vi "Input 信息检测.vi"(9 "Input 配置信息":string[][](table)=[["名称", "点位", "索引号", "逻辑取反"], ["启动按钮", "X100", "0", "0"], ["复位按钮", "X101", "1", "0"], ["暂停按钮", "X102", "2", "0"], ["操作侧安全光栅", "X103", "3", "0"], ["后侧安全光栅", "X104", "4", "0"], ["上层真空检知", "X105", "5", "0"], ["下层真空检知", "X106", "6", "0"], ["上层感应sensor", "X107", "7", "0"], ["下层感应sensor", "X110", "8", "0"], ["传送抓手气缸前位", "X111", "9", "0"], ["传送抓手气缸后位", "X112", "10", "0"], ["上层产品定位气缸前位", "X113", "11", "0"], ["上层产品定位气缸后位", "X114", "12", "0"], ["下层产品定位气缸前位", "X115", "13", "0"], ["下层产品定位气缸后位", "X116", "14", "0"], ["抓手感应产品sensor", "X117", "15", "0"], ["起子1真空检知", "X120", "16", "0"], ["起子2真空检知", "X121", "17", "0"], ["起子3真空检知", "X122", "18", "0"], ["起子4真空检知", "X123", "19", "0"], ["feed01感应sensor", "X124", "20", "0"], ["feed02感应sensor", "X125", "21", "0"], ["feed03感应sensor", "X126", "22", "0"], ["feed04感应sensor", "X127", "23", "0"], ["动子1和2统一坐标sensor", "X130", "24", "0"], ["动子3和4统一坐标sensor", "X131", "25", "0"], ["前后侧统一坐标sensor", "X132", "26", "0"], ["上站允许取料信号", "X133", "27", "0"], ["下站允许投料信号", "X134", "28", "0"], ["上站请求信号", "X135", "29", "0"], ["下站答复信号", "X136", "30", "0"]], 11 "输入读取":T1) -> (2 "Input  ERROR":string[](array[string]))   [LabVIEW 2017]
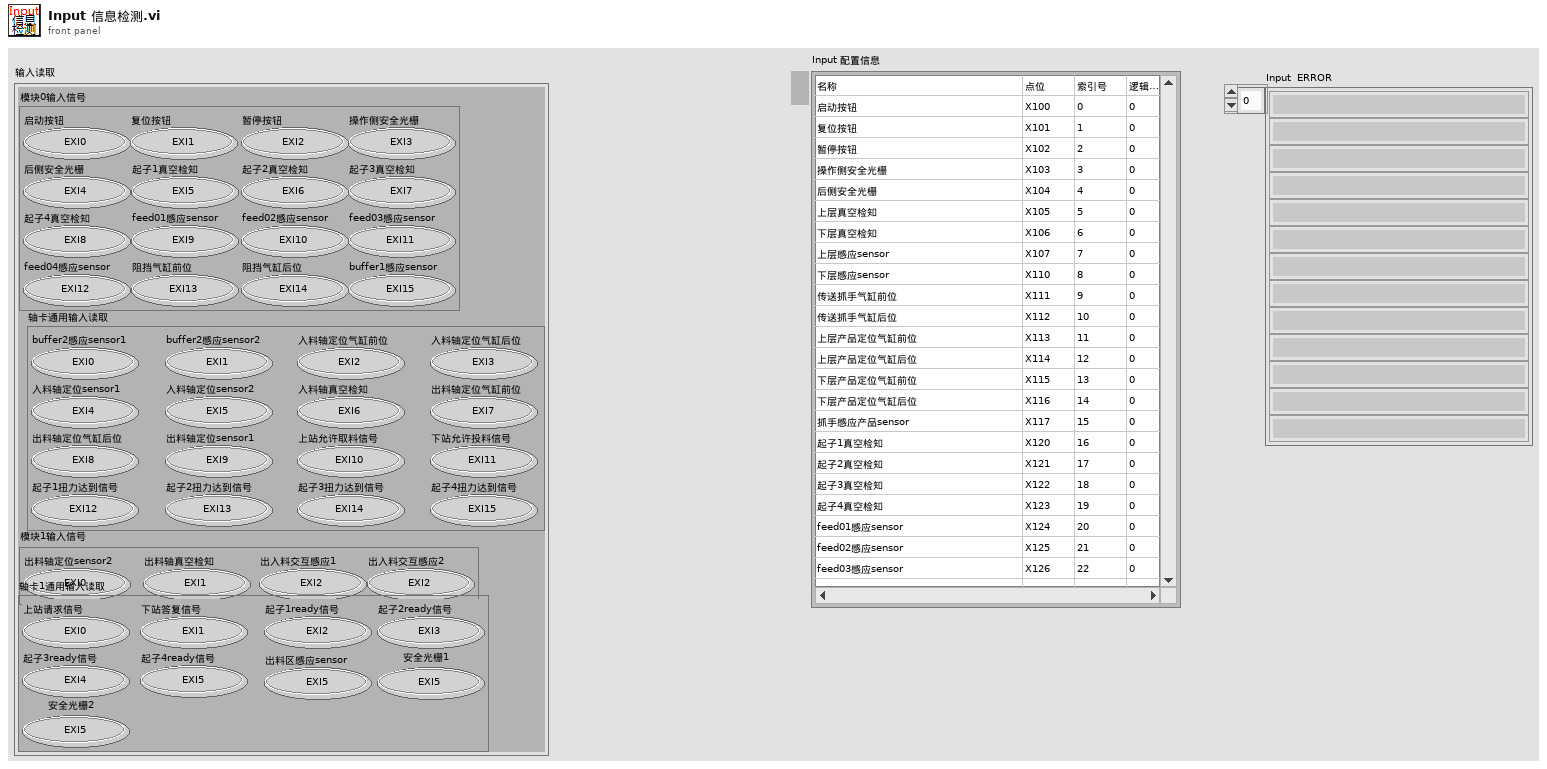
[diagram p1: front panel]
types:
  T1 = typedef "输入读取.ctl" = cluster{"模块0输入信号":T2, "轴卡通用输入读取":T3, "模块1输入信号":T4, "轴卡1通用输入读取":T5}
  T2 = typedef "模块0输入读取.ctl" = cluster{"启动按钮":bool, "复位按钮":bool, "暂停按钮":bool, "操作侧安全光栅":bool, "后侧安全光栅":bool, "起子1真空检知":bool, "起子2真空检知":bool, "起子3真空检知":bool, "起子4真空检知":bool, "feed01感应sensor":bool, "feed02感应sensor":bool, "feed03感应sensor":bool, "feed04感应sensor":bool, "阻挡气缸前位":bool, "阻挡气缸后位":bool, "buffer1感应sensor":bool}
  T3 = typedef "轴卡0通用输入读取.ctl" = cluster{"buffer2感应sensor1":bool, "buffer2感应sensor2":bool, "入料轴定位气缸前位":bool, "入料轴定位气缸后位":bool, "入料轴定位sensor1":bool, "入料轴定位sensor2":bool, "入料轴真空检知":bool, "出料轴定位气缸前位":bool, "出料轴定位气缸后位":bool, "出料轴定位sensor1":bool, "上站允许取料信号":bool, "下站允许投料信号":bool, "起子1扭力达到信号":bool, "起子2扭力达到信号":bool, "起子3扭力达到信号":bool, "起子4扭力达到信号":bool}
  T4 = typedef "模块1输入读取.ctl" = cluster{"出料轴定位sensor2":bool, "出料轴真空检知":bool, "出入料交互感应1":bool, "出入料交互感应2":bool}
  T5 = typedef "轴卡1通用输入读取.ctl" = cluster{"上站请求信号":bool, "下站答复信号":bool, "起子1ready信号":bool, "起子2ready信号":bool, "起子3ready信号":bool, "起子4ready信号":bool, "出料区感应sensor":bool, "安全光栅1":bool, "安全光栅2":bool}
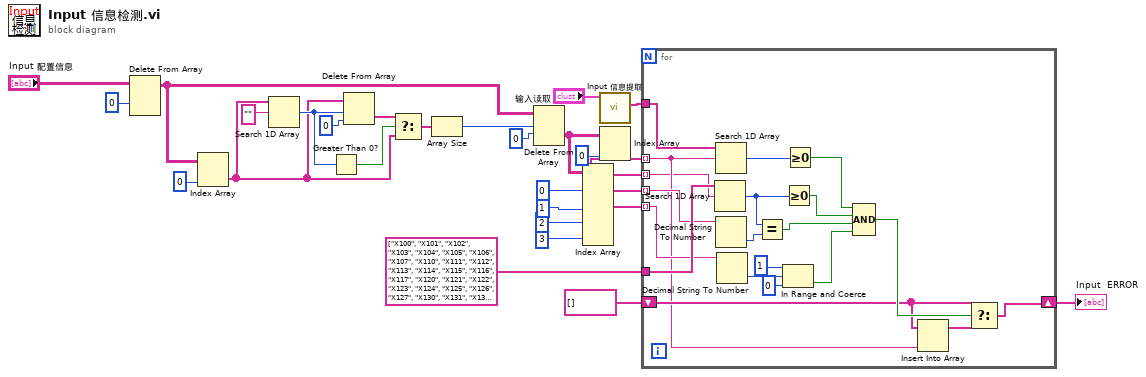
[diagram p0: block diagram]
diagram:
  n1 = Delete From Array(array="Input 配置信息", index (row)=0 ("索引 (行)")) -> (array with subset deleted=w14:string[][])  [unwired: 2 in, 1 out]
  n2 = Index Array(array=w14, index (col)=0 ("禁用的索引 (列)")) -> (element=w17:string[])  [unwired: 1 in]
  n3 = Search 1D Array(1D array=w17, element="") -> (index of element=w21:i32)  [unwired: 1 in]
  n4 = Greater Than 0?(x=w21) -> (x > 0?=w22:bool)
  n5 = Delete From Array(array=w17, length=w21, index=0 ("索引")) -> (deleted portion=w19:string[])  [unwired: 1 out]
  n6 = Select(t=w19, s=w22, f=w17) -> (s? t:f=w16:string[])
  n7 = Array Size(array=w16) -> (size(s)=w18:i32)
  n8 = Delete From Array(array=w14, length=w18, index (row)=0 ("索引 (行)")) -> (deleted portion=w2:string[][])  [unwired: 1 in, 1 out]
  n9 = Index Array(array=w2, index (col) #1=0 ("禁用的索引 (列)"), index (col) #2=1 ("禁用的索引 (列)"), index (col) #3=2 ("禁用的索引 (列)"), index (col) #4=3 ("禁用的索引 (列)")) -> (element #1=w9:string[], element #2=w8:string[], element #3=w7:string[], element #4=w6:string[])  [unwired: 4 in]
  n10 = call "Input 信息提取.vi"("输入读取"="输入读取") -> ("输入读取信号"=w3:string[])  [unwired: 10 in]
  n11 = Index Array(array=w2, index (col)=0 ("禁用的索引 (列)")) -> ()  [unwired: 1 in, 1 out]
  n12 = for {
    tunnel: w9 -> [w30] mode=indexing
    tunnel: w8 -> [w29] mode=indexing
    tunnel: w7 -> [w46] mode=indexing
    tunnel: w6 -> [w43] mode=indexing
    shift-right: [w32] -> w1
    shift-left: string[] [] -> [w34]
    tunnel: string[] ["X100", "X101", "X102", "X103", "X104", "X105", "X106", "X107", "X110", "X111", "X112", "X113", "X114", "X115", "X116", "X117", "X120", "X121", "X122", "X123", "X124", "X125", "X126", "X127", "X130", "X131", "X132", "X133", "X134", "X135", "X136", "X137", "X140", "X141", "X142", "X143", "X144", "X145", "X146", "X147", "X150", "X151", "X152", "X153", "X154", "X155", "X156", "X157", "X160", "X161", "X162", "X163", "X164", "X165", "X166", "X167", "X170", "X171", "X172", "X173", "X174", "X175", "X176", "X177"] ("子数组 2") -> [w47]
    tunnel: w3 -> [w31]
    n13 = Search 1D Array(1D array=w47, element=w29) -> (index of element=w45:i32)  [unwired: 1 in]
    n14 = Search 1D Array(1D array=w31, element=w30) -> (index of element=w48:i32)  [unwired: 1 in]
    n15 = Decimal String To Number(string=w46) -> (number=w44:i32)  [unwired: 2 in, 1 out]
    n16 = Decimal String To Number(string=w43) -> (number=w42:i32)  [unwired: 2 in, 1 out]
    n17 = Equal?(x=w45, y=w44) -> (x = y?=w37:bool)
    n18 = In Range and Coerce(upper limit=1 ("下限"), x=w42, lower limit=0 ("下限")) -> (In Range?=w36:bool)  [unwired: 1 out]
    n19 = Greater Or Equal To 0?(x=w45) -> (x >= 0?=w38:bool)
    n20 = Greater Or Equal To 0?(x=w48) -> (x >= 0?=w39:bool)
    n21 = Compound Arithmetic op=AND(w39, w38, w37, w36) -> (w35:bool)
    n22 = Insert Into Array(array=w34, new element=w30) -> (w33:string[])  [unwired: 1 in]
    n23 = Select(t=w34, s=w35, f=w33) -> (s? t:f=w32:string[])
  }
  "Input  ERROR" <- w1
